vi "image_stitchinf_v2.vi"(9 "Image":T1(plugin-control), 10 "Path 2":path, 11 "Path":path) -> (0 "coloana 2":i32, 1 "RANDU 2":i32, 2 "COLOANA 1":i32, 3 "RANDU 1":i32)   [LabVIEW 2015]
panel:
  out "24-bit pixmap":u32[][](array[numeric]) format="%x"
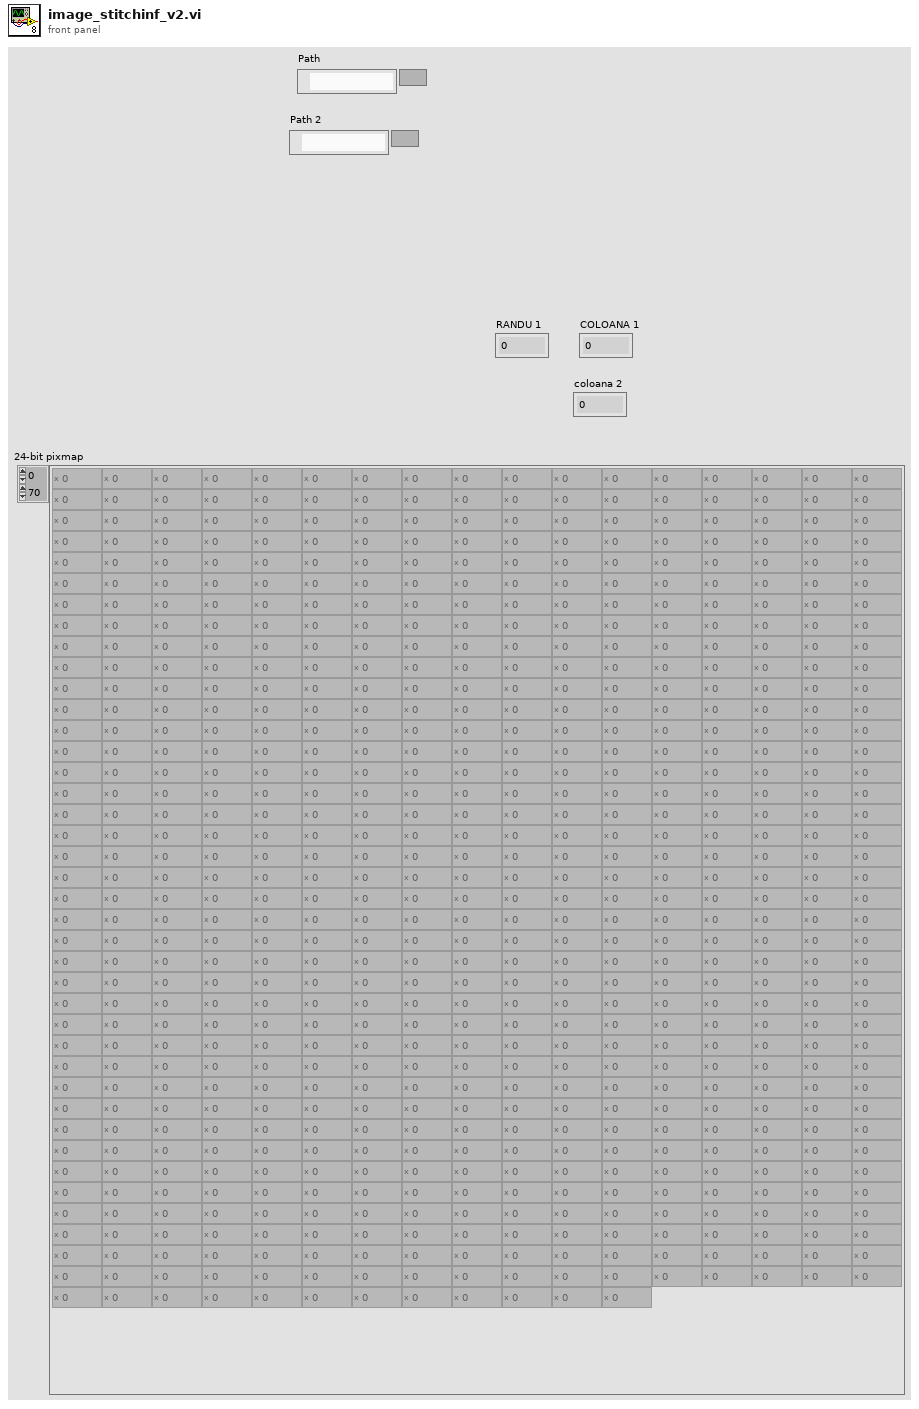
[diagram p1: front panel]
types:
  T1 = typedef "IMAQ Image.ctl" = refnum<image>
  T2 = typedef "imagedata.ctl" = cluster{"image type":i32, "image depth":i32, "image":u8[], "mask":u8[], "colors":u32[], "Rectangle":cluster{"left":i16, "top":i16, "right":i16, "bottom":i16}}
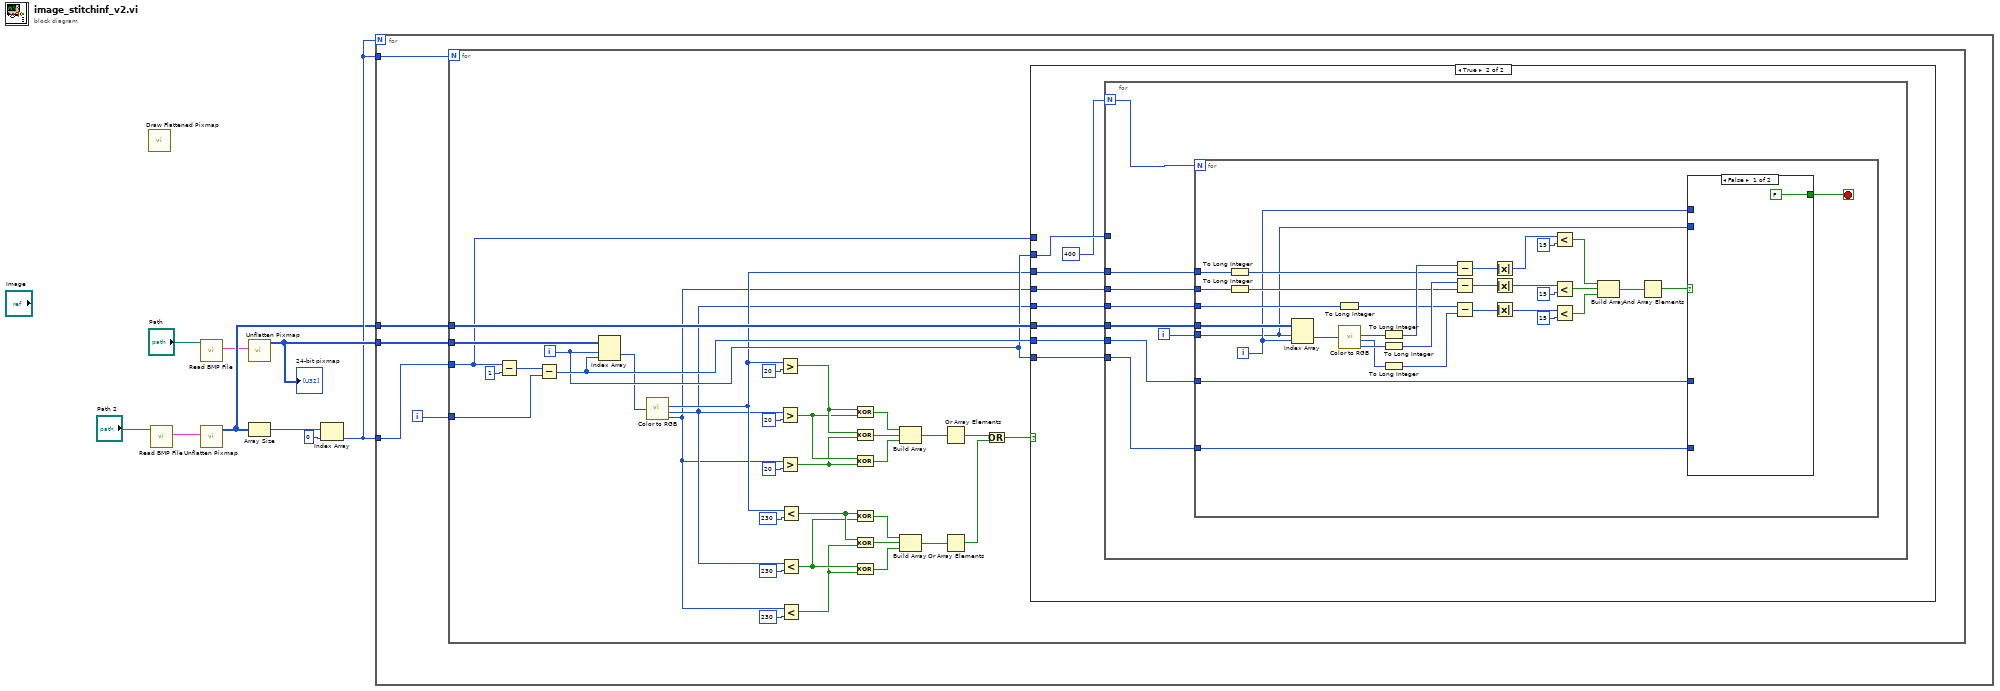
[diagram p0: block diagram]
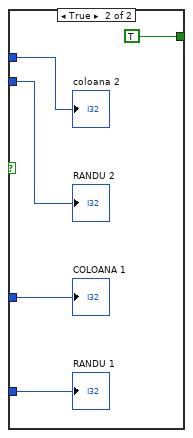
[diagram p3: hidden frame]
diagram:
  n1 = call <vilib>:"Draw Flattened Pixmap.vi"() -> ()  [unwired: 9 in, 1 out]
  n2 = call <vilib>:"Read BMP File.vi"("path to BMP file"="Path 2") -> ("image data"=w3:T2)  [unwired: 8 in, 2 out]
  n3 = call <vilib>:"Read BMP File.vi"("path to BMP file"="Path") -> ("image data"=w1:T2)  [unwired: 8 in, 2 out]
  n4 = call <vilib>:"Unflatten Pixmap.vi"("image data"=w3) -> ("24-bit pixmap"=w5:u32[][])  [unwired: 4 in, 6 out]
  n5 = call <vilib>:"Unflatten Pixmap.vi"("image data"=w1) -> ("24-bit pixmap"=w7:u32[][])  [unwired: 4 in, 6 out]
  "24-bit pixmap" <- w7
  n6 = Array Size(array=w5) -> (size(s)=w9:i32[])
  n7 = Index Array(array=w9, index=0) -> (element=w6:i32)
  n8 = for {
    N: w6 -> [_]
    tunnel: w7 -> [w14]
    tunnel: w6 -> [w13]
    tunnel: w5 -> [w11]
    tunnel: w6 -> [w10]
    i -> [w12]
    n9 = for {
      N: w13 -> [_]
      tunnel: w14 -> [w49]
      tunnel: w12 -> [w40]
      tunnel: w11 -> [w42]
      tunnel: w10 -> [w33]
      i -> [w38]
      n10 = Subtract(x=w33, y=1) -> (x-y=w31:i32)
      n11 = Subtract(x=w31, y=w40) -> (x-y=w39:i32)
      n12 = Index Array(array=w49, index (row)=w38, index (col)=w39) -> (element=w37:u32)
      n13 = call <vilib>:"Color to RGB.vi"("Color"=w37) -> ("R"=w36:u8, "G"=w35:u8, "B"=w34:u8)  [unwired: 1 out]
      n14 = Greater?(x=w36, y=u8 20) -> (0:w18:bool)
      n15 = Greater?(x=w35, y=u8 20) -> (0:w17:bool)
      n16 = Greater?(x=w34, y=u8 20) -> (0:w16:bool)
      n17 = Less?(x=w36, y=u8 230) -> (x < y?=w25:bool)
      n18 = Less?(x=w35, y=u8 230) -> (x < y?=w24:bool)
      n19 = Less?(x=w34, y=u8 230) -> (x < y?=w23:bool)
      n20 = Exclusive Or(1:w17, 2:w18) -> (0:w22:bool)
      n21 = Exclusive Or(1:w16, 2:w18) -> (0:w21:bool)
      n22 = Exclusive Or(1:w16, 2:w17) -> (0:w20:bool)
      n23 = Exclusive Or(1:w24, 2:w25) -> (0:w30:bool)
      n24 = Exclusive Or(1:w23, 2:w25) -> (0:w29:bool)
      n25 = Exclusive Or(1:w23, 2:w24) -> (0:w28:bool)
      n26 = Build Array(w22, w21, w20) -> (w19:bool[])
      n27 = Build Array(w30, w29, w28) -> (w26:bool[])
      n28 = Or Array Elements(Boolean array=w19) -> (logical OR=w15:bool)
      n29 = Or Array Elements(Boolean array=w26) -> (logical OR=w27:bool)
      n30 = Or(x=w15, y=w27) -> (x .or. y?=w41:bool)
      n31 = case shown="True" w41 {
        tunnel: w42 -> [_ w57]
        tunnel: w36 -> [_ w55]
        tunnel: w35 -> [_ w54]
        tunnel: w34 -> [_ w53]
        tunnel: w33 -> [_ _]
        tunnel: w38 -> [_ w56]
        tunnel: w38 -> [_ w52]
        tunnel: w39 -> [_ w51]
        frame False {
        }
        frame True {
          n32 = for {
            N: 400 -> [w58]
            tunnel: w57 -> [w65]
            tunnel: w56 -> [_]
            tunnel: w55 -> [w64]
            tunnel: w54 -> [w63]
            tunnel: w53 -> [w62]
            tunnel: w52 -> [w61]
            tunnel: w51 -> [w60]
            i -> [w59]
            n33 = for {
              N: w58 -> [_]
              tunnel: w65 -> [w98]
              tunnel: w59 -> [w66]
              tunnel: w64 -> [w77]
              tunnel: w63 -> [w76]
              tunnel: w62 -> [w67]
              tunnel: w61 -> [w71]
              tunnel: w60 -> [w70]
              i -> [w73]
              stop <- w72 stop-if-true
              n34 = To Long Integer(number=w77) -> (32bit integer=w96:i32)
              n35 = To Long Integer(number=w67) -> (32bit integer=w93:i32)
              n36 = Index Array(array=w98, index (row)=w66, index (col)=w73) -> (element=w79:u32)
              n37 = To Long Integer(number=w76) -> (32bit integer=w91:i32)
              n38 = call <vilib>:"Color to RGB.vi"("Color"=w79) -> ("R"=w69:u8, "G"=w68:u8, "B"=w78:u8)  [unwired: 1 out]
              n39 = To Long Integer(number=w69) -> (32bit integer=w97:i32)
              n40 = To Long Integer(number=w78) -> (32bit integer=w94:i32)
              n41 = To Long Integer(number=w68) -> (32bit integer=w90:i32)
              n42 = Subtract(x=w97, y=w96) -> (x-y=w95:i32)
              n43 = Subtract(x=w94, y=w93) -> (x-y=w92:i32)
              n44 = Subtract(x=w91, y=w90) -> (x-y=w89:i32)
              n45 = Absolute Value(x=w95) -> (abs(x)=w88:i32)
              n46 = Absolute Value(x=w92) -> (abs(x)=w84:i32)
              n47 = Absolute Value(x=w89) -> (abs(x)=w83:i32)
              n48 = Less?(x=w88, y=15) -> (x < y?=w82:bool)
              n49 = Less?(x=w84, y=15) -> (x < y?=w81:bool)
              n50 = Less?(x=w83, y=15) -> (x < y?=w80:bool)
              n51 = Build Array(w82, w81, w80) -> (w75:bool[])
              n52 = And Array Elements(Boolean array=w75) -> (logical AND=w74:bool)
              n53 = case shown="False" w74 {
                tunnel: w73 -> [_ w104]
                tunnel: [FALSE TRUE] -> w72
                tunnel: w71 -> [_ w102]
                tunnel: w70 -> [_ w101]
                tunnel: w66 -> [_ w100]
                frame False {
                }
                frame True {
                  "coloana 2" <- w104
                  "RANDU 1" <- w102
                  "COLOANA 1" <- w101
                  "RANDU 2" <- w100
                }
              }
            }
          }
        }
      }
    }
  }
